vi "Read Water Level.vi"(11 "Update Water Level Msg in":refnum<class "Update Water Level Msg.lvclass">) -> (2 "Water Level":dbl, 3 "Update Water Level Msg out":refnum<class "Update Water Level Msg.lvclass">)   [LabVIEW 2018, in "Water Level.lvlib" / "Update Water Level Msg.lvclass"]
doc: "Reads the depth of the water in the water basin."
uses:
  Update Water Level Msg.lvclass
  Update Water Level Msg.lvclass/Update Water Level Msg.ctl
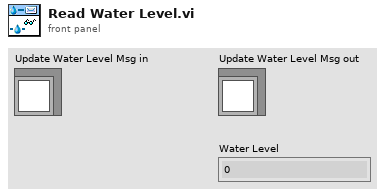
[diagram p1: front panel]
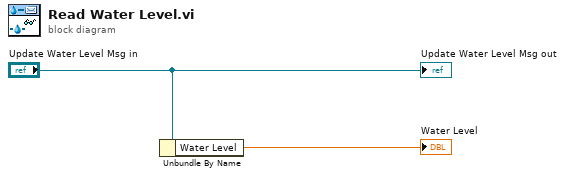
[diagram p0: block diagram]
diagram:
  n1 = Unbundle By Name("Update Water Level Msg in") -> ("Water Level"=→"Water Level":dbl)
  "Update Water Level Msg out" <- "Update Water Level Msg in"
